vi "incoming data.vi"(6 "timeout":i32=-1, 8 "error in":errorcluster, 9 "opcode":u8=1, 10 "data":string, 11 "websocket user plugin in":refnum<class "websocket user plugin.lvclass">) -> (0 "error out":errorcluster)   [LabVIEW 2013, in "websocket user plugin.lvclass"]
uses:
  websocket user plugin.lvclass
  opcode.ctl
  websocket core.lvlib
panel:
  out "opcode 2":T1=1 items=["text"=1, "binary"=2, "x3"=3, "x4"=4, "x5"=5, "x6"=6, "x7"=7]
  out "data 2":string
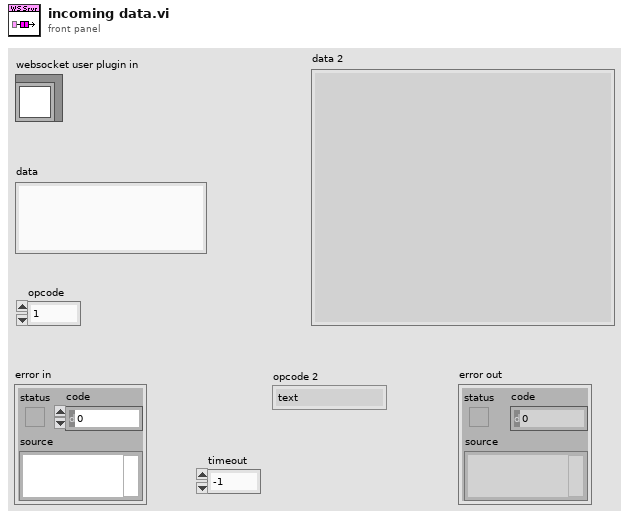
[diagram p1: front panel]
types:
  T1 = typedef "websocket core.lvlib/opcode.ctl" = u8
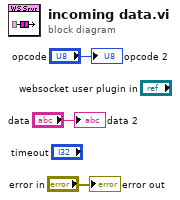
[diagram p0: block diagram]
diagram:
  "error out" <- "error in"
  "data 2" <- "data"
  "opcode 2" <- "opcode"
